vi "remote.Read Dev.VendorNum.vi"(8 "error in (no error)":errorcluster, 11 "SLSC Remote in":refnum<class "SLSC Interface.lvclass">) -> (0 "error out":errorcluster, 2 "Dev.VendorNum":u32, 3 "SLSC Remote out":refnum<class "SLSC Interface.lvclass">)   [LabVIEW 2016, in "SLSC Interfaces.lvlib" / "SLSC Interface.lvclass"]
uses:
  SLSC Interface Class/SLSC Interface.lvclass
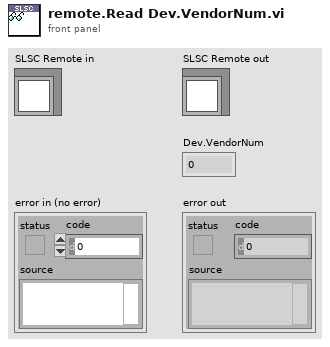
[diagram p1: front panel]
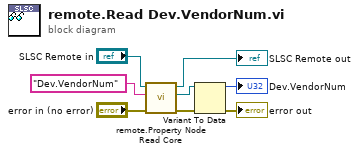
[diagram p0: block diagram]
diagram:
  n1 = call "remote.Property Node Read Core.vi"("error in (no error)"="error in (no error)", "property"="Dev.VendorNum", "SLSC Remote in"="SLSC Remote in") -> ("error out"=w8:errorcluster, "value"=w3:refnum<class "JSON Null.lvclass">, "SLSC Remote out"=→"SLSC Remote out":refnum<class "SLSC Interface.lvclass">)  [unwired: 6 in]
  n2 = Variant To Data(error in=w8, Variant=w3) -> (data=→"Dev.VendorNum":u32, error out=→"error out":errorcluster)  [unwired: 1 in]
